vi "Configure Client.vi"(8 "error in (no error)":errorcluster, 10 "Client in":refnum<class "Connection.lvclass">, 11 "SerialResource in":refnum<class "SerialResource.lvclass">) -> (0 "error out":errorcluster, 2 "Client":refnum<class "Connection.lvclass">, 3 "SerialResource out":refnum<class "SerialResource.lvclass">)   [LabVIEW 2020, in "PicoG-Core.lvlib" / "SerialResource.lvclass"]
uses:
  SerialResource.lvclass
  <vilib>/IlluminatedG/lv-stream/Connection/Connection.lvclass
  SerialResource.lvclass/SerialResource.ctl
  <vilib>/IlluminatedG/IG Serial Stream/Stream-Serial/Serial Client/Serial Client.lvclass
  <vilib>/IlluminatedG/IG Serial Stream/Stream-Serial/Serial Client/Stop Bits.ctl
  <vilib>/IlluminatedG/IG Serial Stream/Stream-Serial/Serial Client/Flow Control.ctl
  <vilib>/IlluminatedG/IG Serial Stream/Stream-Serial/Serial Client/Parity.ctl
  <vilib>/IlluminatedG/IG Serial Stream/Stream-Serial/Serial Client/Port Config.ctl
  <vilib>/IlluminatedG/lv-stream/Endpoint/Endpoint.lvclass
  C:/Program Files (x86)/National Instruments/LabVIEW 2020/vi.lib/IlluminatedG/lv-stream/Connection/Connection.lvclass
  C:/Program Files (x86)/National Instruments/LabVIEW 2020/vi.lib/IlluminatedG/lv-stream/Endpoint/Endpoint.lvclass
  C:/Program Files (x86)/National Instruments/LabVIEW 2020/vi.lib/IlluminatedG/IG Serial Stream/Stream-Serial/Serial Client/Serial Client.lvclass
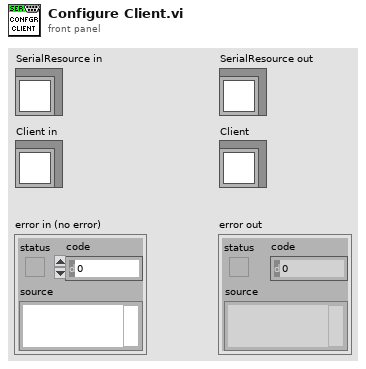
[diagram p1: front panel]
types:
  T1 = typedef "Stream-Serial.lvlib/Serial Client.lvclass/Port Config.ctl" = cluster{"Baud (115200)":u32, "Data Bits (8)":u8, "Stop Bits (1)":T2, "Flow Control":T3, "Use LineTerm?":bool, "LineTerm (\\n)":string, "Timeout ms (10000)":i32, "Parity (None)":T4}
  T2 = typedef "Stream-Serial.lvlib/Serial Client.lvclass/Stop Bits.ctl" = u16
  T3 = typedef "Stream-Serial.lvlib/Serial Client.lvclass/Flow Control.ctl" = u16
  T4 = typedef "Stream-Serial.lvlib/Serial Client.lvclass/Parity.ctl" = enum16{"None", "Odd", "Even", "Mark", "Space"}
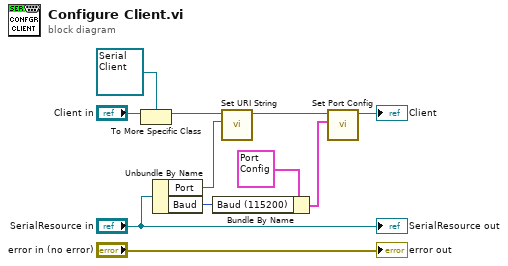
[diagram p0: block diagram]
diagram:
  n1 = To More Specific Class(target class=refnum<class "Serial Client.lvclass"> refnum ("Stream-Serial.lvlib:Serial Client.lvclass"), reference="Client in") -> (specific class reference=w3:refnum<class "Serial Client.lvclass">)  [unwired: 1 in, 1 out]
  n2 = Unbundle By Name("SerialResource in") -> ("Port"=w1:refnum<visa-resource-name>, "Baud"=w6:u32)
  n3 = Bundle By Name(cluster=T1 {"Baud (115200)"=115200, "Data Bits (8)"=8, "Stop Bits (1)"=10, "Flow Control"=0, "Use LineTerm?"=FALSE, "LineTerm (\\n)"="\n", "Timeout ms (10000)"=10000, "Parity (None)"=enum."None"} ("Port Config"), "Baud (115200)"=w6) -> (w5:T1)
  n4 = call <vilib>:"Set URI String.vi"("URI String"=w1, "Endpoint in"=w3) -> ("Endpoint out"=w2:refnum<class "Serial Client.lvclass">)  [unwired: 8 in, 1 out]
  n5 = call <vilib>:"Set Port Config.vi"("Port Config"=w5, "Serial Client in"=w2) -> ("Serial Client out"=→"Client":refnum<class "Serial Client.lvclass">)  [unwired: 8 in, 1 out]
  "error out" <- "error in (no error)"
  "SerialResource out" <- "SerialResource in"
